vi "generate number.vi"(11 "number":dbl format="%#_16g") -> (3 "nunber string":string)   [LabVIEW 2013, in "json generator.lvlib"]
uses:
  json generator.lvlib
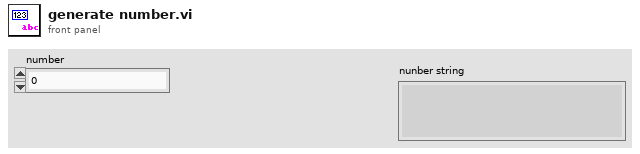
[diagram p1: front panel]
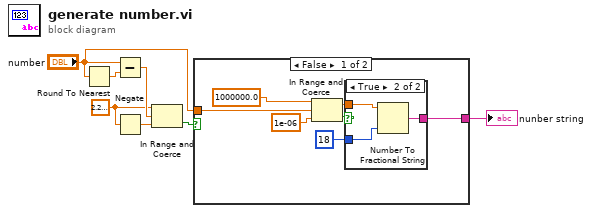
[diagram p0: block diagram]
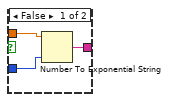
[diagram p2: hidden frame]
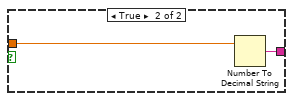
[diagram p3: hidden frame]
diagram:
  w4 = 2.220446049250313e-16
  n1 = Round To Nearest(number="number") -> (nearest integer value=w7:dbl)
  n2 = Subtract(x="number", y=w7) -> (x-y=w6:dbl)
  n3 = Negate(x=w4) -> (-x=w5:dbl)
  n4 = In Range and Coerce(upper limit=w4, x=w6, lower limit=w5) -> (In Range?=w3:bool)  [unwired: 1 out]
  n5 = case shown="False" w3 {
    tunnel: "number" -> [w13 w22]
    tunnel: [w9 w21] -> w2
    frame False {
      n6 = In Range and Coerce(upper limit=1000000.0, x=w13, lower limit=1e-06) -> (coerced(x)=w10:dbl, In Range?=w14:bool)
      n7 = case shown="True" w14 {
        tunnel: w10 -> [w17 w20]
        tunnel: [w16 w19] -> w9
        tunnel: i16 18 ("precision (6)") -> [w15 w18]
        frame False {
          n8 = Number To Exponential String(number=w17, precision (6)=w15) -> (E-format string=w16:string)  [unwired: 2 in]
        }
        frame True {
          n9 = Number To Fractional String(number=w20, precision (6)=w18) -> (F-format string=w19:string)  [unwired: 2 in]
        }
      }
    }
    frame True {
      n10 = Number To Decimal String(number=w22) -> (decimal integer string=w21:string)  [unwired: 1 in]
    }
  }
  "nunber string" <- w2
